vi "Viewer wrapper.vi"() -> ()   [LabVIEW 2015]
uses:
  User Interface/Viewer/Viewer.lvclass
  <vilib>/ActorFramework/Actor/Actor.lvclass
  <vilib>/ActorFramework/Stop Msg/Stop Msg.lvclass
  GLOBAL/GLOBAL Time-critical.vi
  <vilib>/Analysis/NI_AALBase.lvlib
panel:
  in  "Height":i32=256
  in  "Width":i32=256
  in  "Timeout (ms)":i32=100
  in  "Stop":bool
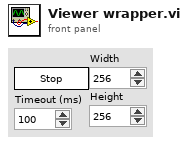
[diagram p1: front panel]
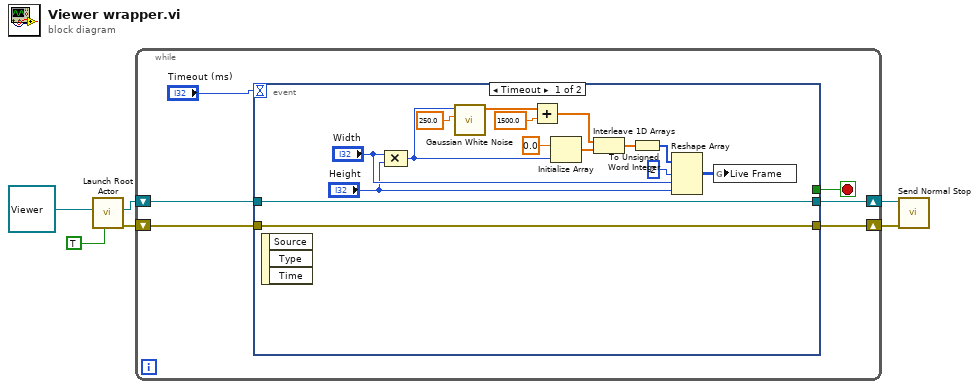
[diagram p0: block diagram]
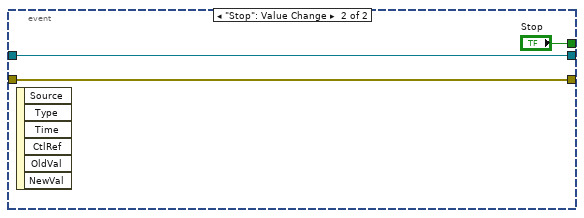
[diagram p2: hidden frame]
diagram:
  n1 = call <vilib>:"Launch Root Actor.vi"("Open Actor Core front panel? (F)"=TRUE, "Actor"=refnum<class "Viewer.lvclass"> refnum ("Viewer.lvlib:Viewer.lvclass")) -> ("error out"=w2:errorcluster, "Actor's Enqueuer"=w4:refnum<class "Message Enqueuer.lvclass">)  [unwired: 8 in]
  n2 = while {
    shift-right: [w11] -> w3
    shift-left: w4 -> [w12]
    shift-right: [w9] -> w1
    shift-left: w2 -> [w10]
    stop <- w8 stop-if-true
    n3 = event shown="[0] Timeout" {
      selector: _ -> [_ _]
      dyn-events: _ -> [_ _]
      timeout: "Timeout (ms)" -> [_ _]
      tunnel: w12 -> [w21 w30]
      tunnel: [w21 w30] -> w11
      tunnel: w10 -> [w22 w29]
      tunnel: [w22 w29] -> w9
      tunnel: [_ "Stop"] -> w8
      event Timeout {
        n4 = event-data() -> ()  [unwired: 1 in, 3 out]
        n5 = Compound Arithmetic op=MULTIPLY("Width", "Height") -> (w17:i32)
        n6 = call <vilib>:"Gaussian White Noise.vi"("standard deviation"=250.0, "samples"=w17) -> ("Gaussian noise pattern"=w18:dbl[])  [unwired: 8 in, 1 out]
        n7 = Add(x=w18, y=1500.0) -> (x+y=w15:dbl[])
        n8 = Initialize Array(0.0 ("element"), w17) -> (w14:dbl[])
        n9 = Interleave 1D Arrays(w15, w14) -> (w13:dbl[])
        n10 = To Unsigned Word Integer(number=w13) -> (unsigned 16bit integer=w24:u16[])
        n11 = Reshape Array(w24, 2 ("value"), "Width", "Height") -> (w23:u16[][][])
        n12 = global write "GLOBAL Time-critical.vi" "Live Frame"(w23) -> ()
      }
      event "Stop": Value Change {
        n13 = event-data() -> ()  [unwired: 1 in, 6 out]
      }
    }
  }
  n14 = call <vilib>:"Send Normal Stop.vi"("error in (no error)"=w1, "Message Enqueuer"=w3) -> ()  [unwired: 9 in, 1 out]
